vi "UMLEditor ToolBarSettings.vi"(1 "localVariables":T3 {"ObjectHotspots"."HotSpot"."y" format="%.2f"; "ObjectHotspots"."HotSpot"."x" format="%.2f"; "NodesBounds"."height" format="%.2f"; "NodesBounds"."width" format="%.2f"; "NodesBounds"."y" format="%.2f"; "NodesBounds"."x" format="%.2f"; "offset"."y" format="%.2f"; "offset"."x" format="%.2f"; "gridSize" format="%.2f"; "dragStartBounds"."height" format="%.2f"; "dragStartBounds"."width" format="%.2f"; "dragStartBounds"."y" format="%.2f"; "dragStartBounds"."x" format="%.2f"; "dragStartPoint"."y" format="%.2f"; "dragStartPoint"."x" format="%.2f"; "rubberBandStart"."y" format="%.2f"; "rubberBandStart"."x" format="%.2f"; "lastMousePoint"."y" format="%.2f"; "lastMousePoint"."x" format="%.2f"; "zoom" format="%.2f"}, 2 "NodeName/EdgeName(empty=not in use)":string, 3 "graph(only used with className input)":refnum<class "Graph.lvclass">, 5 "error in (no error)":errorcluster) -> (14 "diagramType":string, 15 "toolType":T2, 16 "tools":T1, 17 "prototypeEdge":refnum<class "AbstractEdge.lvclass">, 18 "prototypeNode":refnum<class "AbstractNode.lvclass">, 19 "error out":errorcluster)   [LabVIEW 2014]
doc: "Get Tollbar info\nif NodeName/EdgeName is used ..."
uses:
  <resource>/Framework/Providers/Open_GDS/UML/UMLEditor/UMLEditor LocalVariablesType.ctl
  <resource>/Framework/Providers/Open_GDS/UML/AbstractNode_class/AbstractNode.lvclass
  <resource>/Framework/Providers/Open_GDS/UML/AbstractEdge_class/AbstractEdge.lvclass
  <resource>/Framework/Providers/Open_GDS/UML/Graphics_class/Graphics.lvclass
  <resource>/Framework/Providers/Open_GDS/UML/Grid_class/Grid.lvclass
  <resource>/Framework/Providers/Open_GDS/UML/UMLEditor/UMLEditor statesType.ctl
  <resource>/Framework/Providers/Open_GDS/UML/UMLEditor/UMLEditor tooltype.ctl
  <resource>/Framework/Providers/Open_GDS/UML/UMLEditor/UMLEditor toolsType.ctl
  <resource>/Framework/Providers/Open_GDS/UML/UMLEditor/UMLEditor_DiagramInfo.ctl
  <resource>/Framework/Providers/Open_GDS/UML/Graph_class/Graph.lvclass
  <resource>/Framework/Providers/Open_GDS/UML/General/Point/Point Point2D.ctl
  <resource>/Framework/Providers/Open_GDS/UML/General/Rectangle/Rectangle Rectangle2D.ctl
  <resource>/Framework/Providers/Open_GDS/UML/UMLEditor/UMLEditor ExportType.ctl
  <resource>/Framework/Providers/Open_GDS/UML/UMLEditor/UMLEditor FlattenCommandType.ctl
  <resource>/Framework/Providers/Open_GDS/UML/UMLEditor/UMLEditor ExecuteCommandType.ctl
  <resource>/Framework/Providers/Open_GDS/UML/ContextHelp/ContextHelp_EventType.ctl
  <resource>/Framework/Providers/Open_GDS/UML/UMLEditor/UMLEditor_HotSpotData.ctl
  <resource>/Framework/Providers/Open_GDS/UML/UMLEditor/UMLEditor_HotSpotType.ctl
  <resource>/Framework/Providers/Open_GDS/UML/UmlEditor_class/EventData.ctl
  <resource>/Framework/Providers/Open_GDS/UML/UMLEditor/UMLEditor_DiagramType.ctl
  <resource>/Framework/Providers/Open_GDS/UML/UmlEditor_class/UmlEditor.lvclass
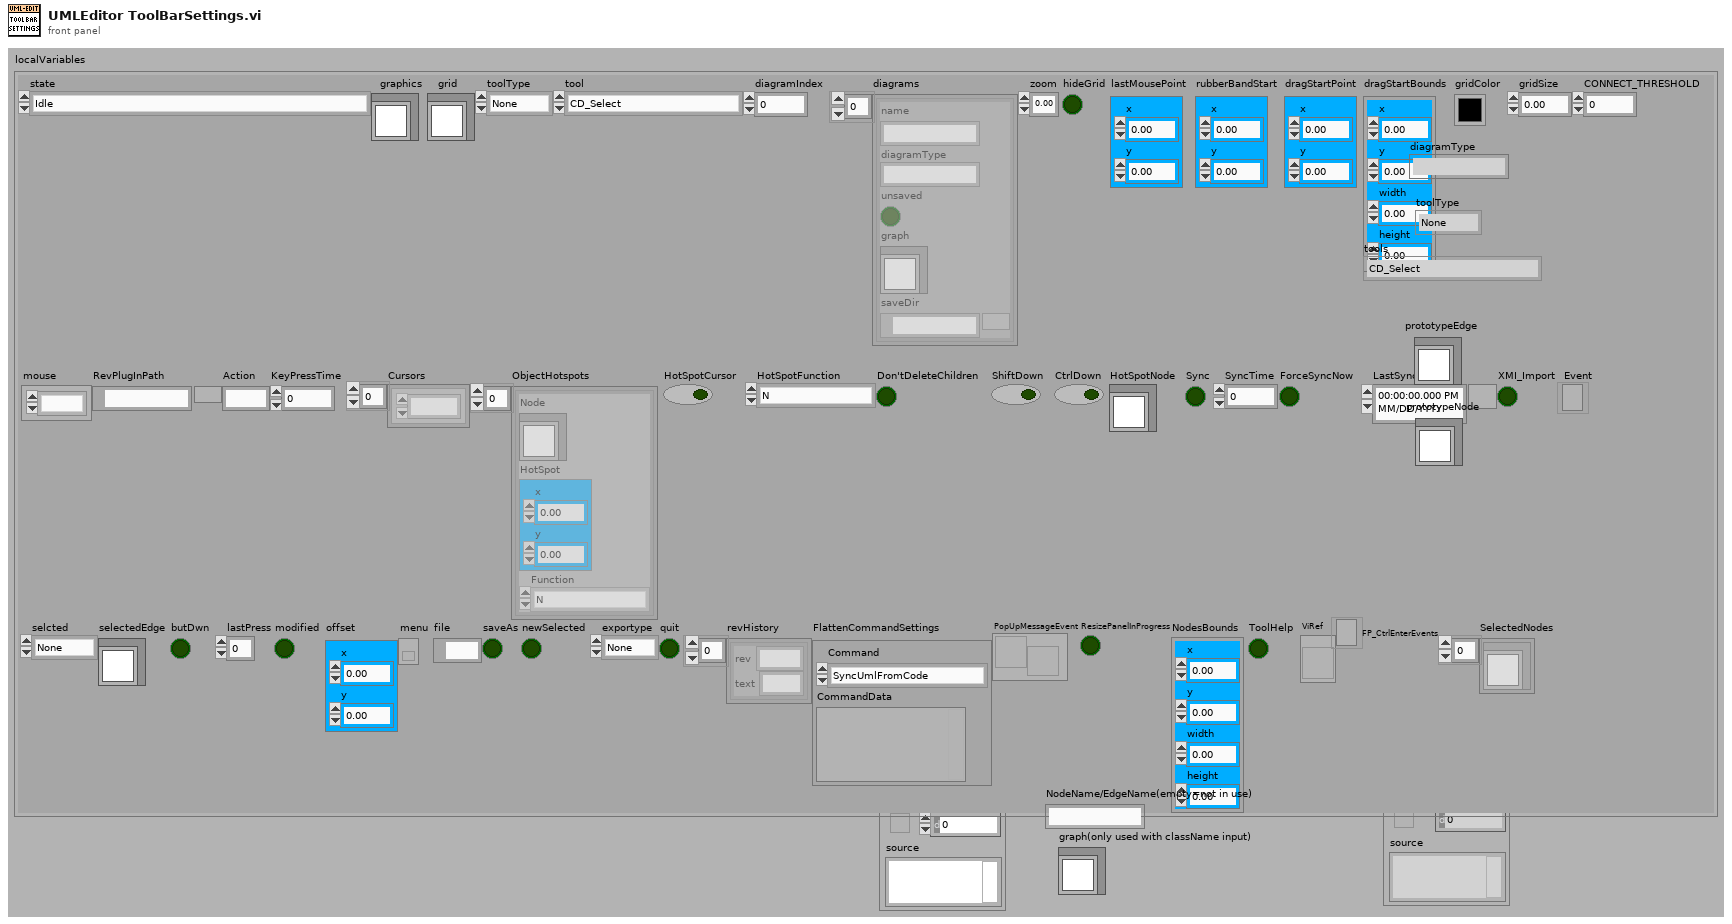
[diagram p1: front panel]
types:
  T1 = typedef "UMLEditor toolsType.ctl" = enum16{"CD_Select", "CD_Class", "CD_Interface", "CD_Package", "CD_Note", "CD_Dependency", "CD_Inheritance", "CD_InterfaceImp", "CD_Association", "CD_Aggregation", "CD_Composite", "CD_NoteConn", "SQD_Select", "SQD_Object", "SQD_ActionBar", "SQD_Note", "SQD_Call", "SQD_NoteConn", "UD_Select", "UD_System", "UD_Actor", "UD_UseCase", "UD_Note", "UD_Assoiciation", "UD_Generalization", "UD_GeneralizationIncludes", "UD_GeneralizationExtends", "UD_Realization", "UD_Relationship", "UD_NoteEdge", "STD_Select", "STD_State", "STD_InitailState", "STD_FinalState", "STD_ChoiseState", "STD_StateTransation", "STD_Note", "STD_NoteEdge", "DM_Select", "DM_VI", "DM_Module", "DM_Request", "DM_RequestWait", "DM_Roundtrip", "DM_Broadcast", "DM_Note", "DM_NoteEdge"}
  T2 = typedef "UMLEditor tooltype.ctl" = enum16{"None", "Node", "Edge"}
  T3 = typedef "UMLEditor LocalVariablesType.ctl" = cluster{"state":T4, "graphics":refnum<class "Graphics.lvclass">, "grid":refnum<class "Grid.lvclass">, "toolType":T2, "tool":T1, "diagramIndex":i32, "diagrams":T5[], "zoom":dbl, "hideGrid":bool, "lastMousePoint":T6, "rubberBandStart":T6, "dragStartPoint":T6, "dragStartBounds":T7, "gridColor":u32, "gridSize":dbl, "CONNECT_THRESHOLD":i32, "selcted":T2, "selectedEdge":refnum<class "AbstractEdge.lvclass">, "butDwn":bool, "lastPress":u32, "modified":bool, "offset":T6, "menu":refnum<k9>, "file":path, "saveAs":bool, "newSelected":bool, "exportype":T8, "quit":bool, "revHistory":cluster{"rev":string, "text":string}[], "FlattenCommandSettings":T9, "PopUpMessageEvent":T11, "ResizePanelInProgress":bool, "NodesBounds":T7, "ToolHelp":bool, "ViRef":refnum<vi>, "FP_CtrlEnterEvents":refnum<event-registration>, "SelectedNodes":refnum<class "AbstractNode.lvclass">[], "mouse":refnum<k1>, "RevPlugInPath":path, "Action":string, "KeyPressTime":u32, "Cursors":refnum<k1>[], "ObjectHotspots":T12[], "HotSpotCursor":bool, "HotSpotFunction":T13, "Don'tDeleteChildren":bool, "ShiftDown":bool, "CtrlDown":bool, "HotSpotNode":refnum<class "AbstractNode.lvclass">, "Sync":bool, "SyncTime":u32, "ForceSyncNow":bool, "LastSync":timestamp, "XMI_Import":bool, "Event":refnum<event-registration>}
  T4 = typedef "UMLEditor statesType.ctl" = enum16{"Idle", "CheckLicense", "revHistory", "Init", "Init2", "EditSelected", "RemoveSelected", "PaintComponent", "ChangeZoom", "ChangeGridSize", "Open", "Close", "Save", "ExportPicture", "Export", "Repaint", "Error", "Exit", "QUIT", "CreateScript", "ExecuteScript", "ClassReversedEngineering", "PlugInReverseEngineering", "StateReversedEngineering", "AutoPlace", "ExecuteCommand", "OpenClass", "SyncAll", "StraightenAssociation", "Copy", "Paste", "AddNodeFromProjectTree", "AddNodeFromProjectTree+SyncAll", "PanAndRepaint", "Init3", "CopyPaste", "ApplyDesignPattern", "AnalyseViInStateDiagram", "AutoSync"}
  T5 = typedef "UMLEditor_DiagramInfo.ctl" = cluster{"name":string, "diagramType":string, "unsaved":bool, "graph":refnum<class "Graph.lvclass">, "saveDir":path}
  T6 = typedef "Point Point2D.ctl" = cluster{"x":dbl, "y":dbl}
  T7 = typedef "Rectangle Rectangle2D.ctl" = cluster{"x":dbl, "y":dbl, "width":dbl, "height":dbl}
  T8 = typedef "UMLEditor ExportType.ctl" = enum16{"None", "Printer", "png", "jpg", "roseUML"}
  T9 = typedef "UMLEditor FlattenCommandType.ctl" = cluster{"Command":T10, "CommandData":variant}
  T10 = typedef "UMLEditor ExecuteCommandType.ctl" = enum16{"SyncUmlFromCode", "SyncCodeFromUML", "OpenClass", "OpenFile", "CreateClass", "CreateVI", "OpenClassAttribute", "LocateInProject"}
  T11 = typedef "ContextHelp_EventType.ctl" = refnum<user-event>
  T12 = typedef "UMLEditor_HotSpotData.ctl" = cluster{"Node":refnum<class "AbstractNode.lvclass">, "HotSpot":T6, "Function":T13}
  T13 = typedef "UMLEditor_HotSpotType.ctl" = enum16{"N", "NE", "E", "SE", "S", "SW", "W", "NW", "Expand", "Collaps"}
  T14 = typedef "UMLEditor_DiagramType.ctl" = string
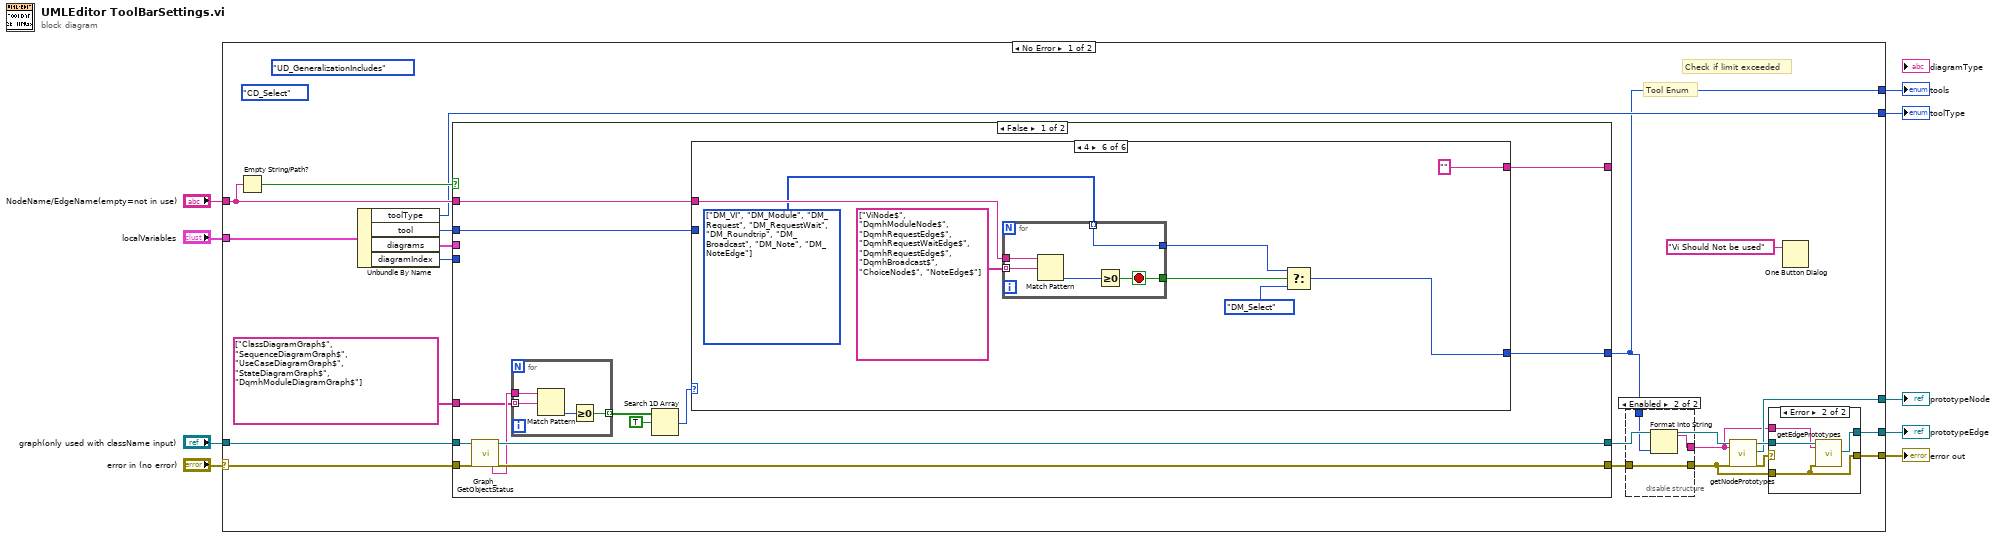
[diagram p0: block diagram]
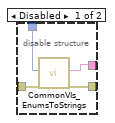
[diagram p2: hidden frame]
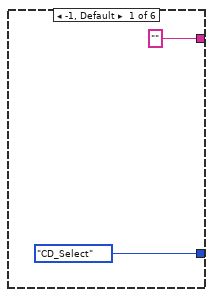
[diagram p4: hidden frame]
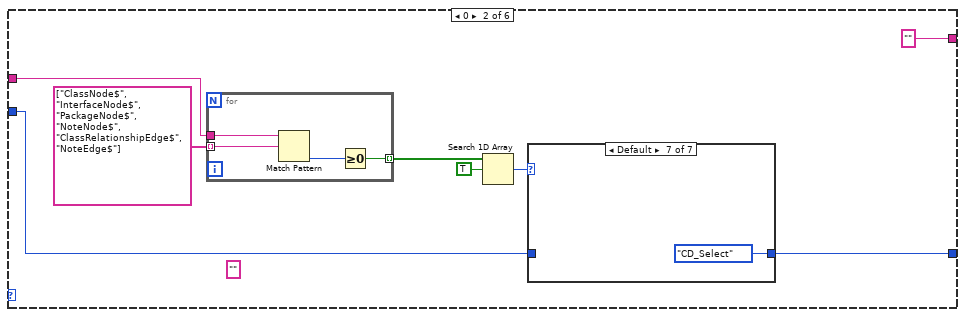
[diagram p5: hidden frame]
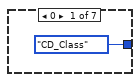
[diagram p6: hidden frame]
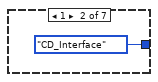
[diagram p7: hidden frame]
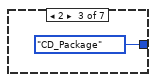
[diagram p8: hidden frame]
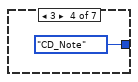
[diagram p9: hidden frame]
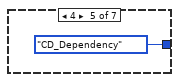
[diagram p10: hidden frame]
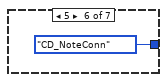
[diagram p11: hidden frame]
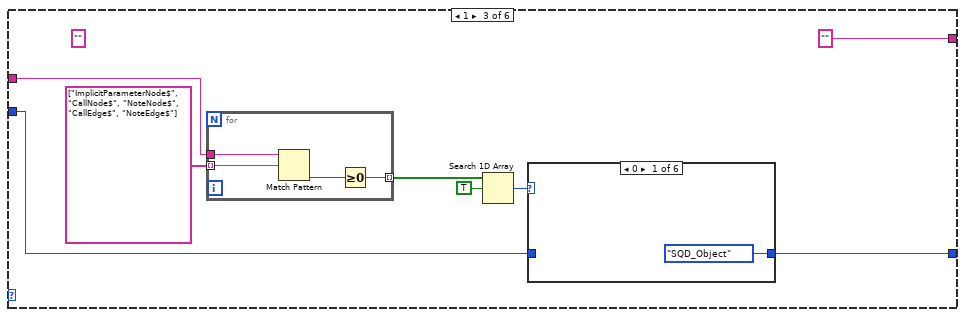
[diagram p12: hidden frame]
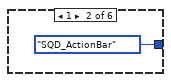
[diagram p13: hidden frame]
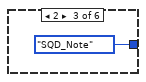
[diagram p14: hidden frame]
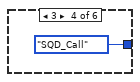
[diagram p15: hidden frame]
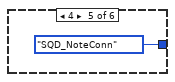
[diagram p16: hidden frame]
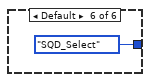
[diagram p17: hidden frame]
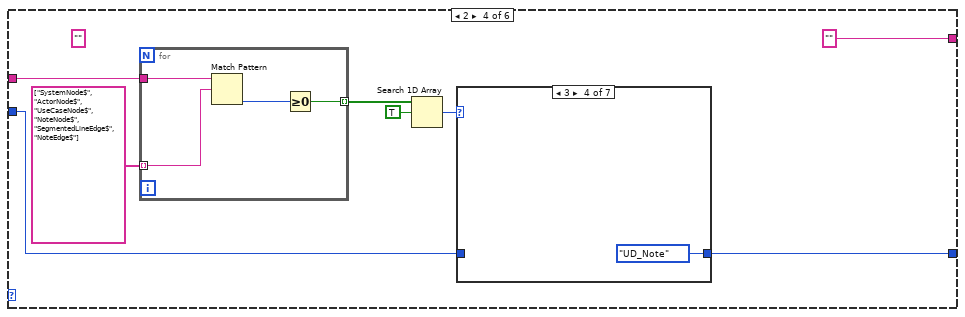
[diagram p18: hidden frame]
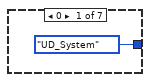
[diagram p19: hidden frame]
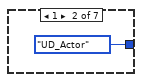
[diagram p20: hidden frame]
diagram:
  n1 = case shown="No Error" "error in (no error)" {
    selector: "error in (no error)" -> [w23 w156]
    tunnel: [w26 w156] -> w8
    tunnel: "localVariables" -> [w14 _]
    tunnel: [w19 _] -> w1
    tunnel: [w15 _] -> w6
    tunnel: [w12 _] -> w5
    tunnel: [w13 _] -> w4
    tunnel: "NodeName/EdgeName(empty=not in use)" -> [w21 _]
    tunnel: "graph(only used with className input)" -> [w24 _]
    frame No Error {
      (unwired) UMLEditor_toolsType."UD_GeneralizationIncludes" ("tool")
      (unwired) UMLEditor_toolsType."CD_Select" ("tool")
      # "Check if limit exceeded"
      # "Tool Enum"
      n2 = Empty String/Path?(string/path=w21) -> (empty?=w22:bool)
      n3 = Unbundle By Name(w14) -> ("toolType"=w13:T2, "tool"=w25:T1, "diagrams"=w30:T5[], "diagramIndex"=w29:i32)
      n4 = case shown="False" w22 {
        tunnel: w30 -> [_ w154]
        tunnel: w29 -> [_ w153]
        tunnel: [w50 w152] -> w28
        tunnel: [w45 _] -> _
        tunnel: w25 -> [w55 w151]
        tunnel: [w54 w151] -> w12
        tunnel: w24 -> [w53 _]
        tunnel: w23 -> [w52 w150]
        tunnel: [w51 w150] -> w18
        tunnel: w21 -> [w49 _]
        tunnel: string[] ["ClassDiagramGraph$", "SequenceDiagramGraph$", "UseCaseDiagramGraph$", "StateDiagramGraph$", "DqmhModuleDiagramGraph$"] -> [w47 _]
        frame False {
          n5 = call <resource>:"Graph_GetObjectStatus.vi"("reference in"=w53, "error in (no error)"=w52) -> ("Class name"=w48:string, "reference out"=w50:refnum<class "Graph.lvclass">, "error out"=w51:errorcluster)  [unwired: 15 out]
          n6 = for {
            tunnel: w48 -> [w149]
            tunnel: w47 -> [w148] mode=indexing
            tunnel: [w146] -> w44 mode=indexing
            n7 = Match Pattern(string=w149, regular expression=w148) -> (offset past match=w147:i32)  [unwired: 4 out]
            n8 = Greater Or Equal To 0?(x=w147) -> (x >= 0?=w146:bool)
          }
          n9 = Search 1D Array(1D array=w44, element=TRUE) -> (index of element=w46:i32)  [unwired: 1 out]
          n10 = case shown="4" w46 {
            tunnel: w55 -> [_ w65 w84 w102 w121 _]
            tunnel: [UMLEditor_toolsType."CD_Select" ("tool") w64 w83 w101 w120 w135] -> w54
            tunnel: w49 -> [_ w62 w81 w99 w118 w139]
            tunnel: [T14 "" ("diagramType") T14 "" ("diagramType") T14 "" ("diagramType") T14 "" ("diagramType") T14 "" ("diagramType") T14 "" ("diagramType")] -> w45
            frame -1, Default {
            }
            frame 0 {
              (unwired) T14 "" ("diagramType")
              n11 = for {
                tunnel: w62 -> [w69]
                tunnel: [w66] -> w59 mode=indexing
                tunnel: string[] ["ClassNode$", "InterfaceNode$", "PackageNode$", "NoteNode$", "ClassRelationshipEdge$", "NoteEdge$"] -> [w68] mode=indexing
                n12 = Match Pattern(string=w69, regular expression=w68) -> (offset past match=w67:i32)  [unwired: 4 out]
                n13 = Greater Or Equal To 0?(x=w67) -> (x >= 0?=w66:bool)
              }
              n14 = Search 1D Array(1D array=w59, element=TRUE) -> (index of element=w58:i32)  [unwired: 1 out]
              n15 = case shown="Default" w58 {
                tunnel: w65 -> [_ _ _ _ _ _ _]
                tunnel: [UMLEditor_toolsType."CD_Class" ("tool") UMLEditor_toolsType."CD_Interface" ("tool") UMLEditor_toolsType."CD_Package" ("tool") UMLEditor_toolsType."CD_Note" ("tool") UMLEditor_toolsType."CD_Dependency" ("tool") UMLEditor_toolsType."CD_NoteConn" ("tool") UMLEditor_toolsType."CD_Select" ("tool")] -> w64
                frame 0 {
                }
                frame 1 {
                }
                frame 2 {
                }
                frame 3 {
                }
                frame 4 {
                }
                frame 5 {
                }
                frame Default {
                }
              }
            }
            frame 1 {
              (unwired) T14 "" ("diagramType")
              n16 = for {
                tunnel: w81 -> [w88]
                tunnel: [w85] -> w78 mode=indexing
                tunnel: string[] ["ImplicitParameterNode$", "CallNode$", "NoteNode$", "CallEdge$", "NoteEdge$"] -> [w87] mode=indexing
                n17 = Match Pattern(string=w88, regular expression=w87) -> (offset past match=w86:i32)  [unwired: 4 out]
                n18 = Greater Or Equal To 0?(x=w86) -> (x >= 0?=w85:bool)
              }
              n19 = Search 1D Array(1D array=w78, element=TRUE) -> (index of element=w77:i32)  [unwired: 1 out]
              n20 = case shown="0" w77 {
                tunnel: w84 -> [_ _ _ _ _ _]
                tunnel: [UMLEditor_toolsType."SQD_Object" ("tool") UMLEditor_toolsType."SQD_ActionBar" ("tool") UMLEditor_toolsType."SQD_Note" ("tool") UMLEditor_toolsType."SQD_Call" ("tool") UMLEditor_toolsType."SQD_NoteConn" ("tool") UMLEditor_toolsType."SQD_Select" ("tool")] -> w83
                frame 0 {
                }
                frame 1 {
                }
                frame 2 {
                }
                frame 3 {
                }
                frame 4 {
                }
                frame Default {
                }
              }
            }
            frame 2 {
              (unwired) T14 "" ("diagramType")
              n21 = for {
                tunnel: w99 -> [w106]
                tunnel: [w103] -> w96 mode=indexing
                tunnel: string[] ["SystemNode$", "ActorNode$", "UseCaseNode$", "NoteNode$", "SegmentedLineEdge$", "NoteEdge$"] -> [w105] mode=indexing
                n22 = Match Pattern(string=w106, regular expression=w105) -> (offset past match=w104:i32)  [unwired: 4 out]
                n23 = Greater Or Equal To 0?(x=w104) -> (x >= 0?=w103:bool)
              }
              n24 = Search 1D Array(1D array=w96, element=TRUE) -> (index of element=w95:i32)  [unwired: 1 out]
              n25 = case shown="3" w95 {
                tunnel: w102 -> [_ _ _ _ _ _ _]
                tunnel: [UMLEditor_toolsType."UD_System" ("tools") UMLEditor_toolsType."UD_Actor" ("tools") UMLEditor_toolsType."UD_UseCase" ("tools") UMLEditor_toolsType."UD_Note" ("tools") UMLEditor_toolsType."UD_Assoiciation" ("tools") UMLEditor_toolsType."UD_NoteEdge" ("tools") UMLEditor_toolsType."UD_Select" ("tool")] -> w101
                frame 0 {
                }
                frame 1 {
                }
                frame 2 {
                }
                frame 3 {
                }
                frame 4 {
                }
                frame 5 {
                }
                frame Default {
                }
              }
            }
            frame 3 {
              (unwired) T14 "" ("diagramType")
              # "NOT IS USE???"
              n26 = for {
                tunnel: w118 -> [w125]
                tunnel: [w122] -> w115 mode=indexing
                tunnel: string[] ["FinalStateNode$", "InitialStateNode$", "StateNode$", "StateTransitionEdge$", "NoteNode$", "NoteEdge$", "ChoiceNode$"] -> [w124] mode=indexing
                n27 = Match Pattern(string=w125, regular expression=w124) -> (offset past match=w123:i32)  [unwired: 4 out]
                n28 = Greater Or Equal To 0?(x=w123) -> (x >= 0?=w122:bool)
              }
              n29 = Search 1D Array(1D array=w115, element=TRUE) -> (index of element=w114:i32)  [unwired: 1 out]
              n30 = case shown="Default" w114 {
                tunnel: w121 -> [_ _ _ _ _ _ _]
                tunnel: [UMLEditor_toolsType."STD_FinalState" ("tools") UMLEditor_toolsType."STD_InitailState" ("tools") UMLEditor_toolsType."STD_State" ("tools") UMLEditor_toolsType."STD_StateTransation" ("tools") UMLEditor_toolsType."STD_Note" ("tools") UMLEditor_toolsType."STD_NoteEdge" ("tools") UMLEditor_toolsType."STD_ChoiseState" ("tools")] -> w120
                frame 0 {
                }
                frame 1 {
                }
                frame 2 {
                }
                frame 3 {
                }
                frame 4 {
                }
                frame Default {
                }
                frame 6 {
                }
              }
            }
            frame 4 {
              w134 = T1[] [enum."DM_VI", enum."DM_Module", enum."DM_Request", enum."DM_RequestWait", enum."DM_Roundtrip", enum."DM_Broadcast", enum."DM_Note", enum."DM_NoteEdge"] items=["CD_Select", "CD_Class", "CD_Interface", "CD_Package", "CD_Note", "CD_Dependency", "CD_Inheritance", "CD_InterfaceImp", "CD_Association", "CD_Aggregation", "CD_Composite", "CD_NoteConn", "SQD_Select", "SQD_Object", "SQD_ActionBar", "SQD_Note", "SQD_Call", "SQD_NoteConn", "UD_Select", "UD_System", "UD_Actor", "UD_UseCase", "UD_Note", "UD_Assoiciation", "UD_Generalization", "UD_GeneralizationIncludes", "UD_GeneralizationExtends", "UD_Realization", "UD_Relationship", "UD_NoteEdge", "STD_Select", "STD_State", "STD_InitailState", "STD_FinalState", "STD_ChoiseState", "STD_StateTransation", "STD_Note", "STD_NoteEdge", "DM_Select", "DM_VI", "DM_Module", "DM_Request", "DM_RequestWait", "DM_Roundtrip", "DM_Broadcast", "DM_Note", "DM_NoteEdge"]
              n31 = for {
                tunnel: w139 -> [w145]
                tunnel: [w142] -> w137
                tunnel: string[] ["ViNode$", "DqmhModuleNode$", "DqmhRequestEdge$", "DqmhRequestWaitEdge$", "DqmhRequestEdge$", "DqmhBroadcast$", "ChoiceNode$", "NoteEdge$"] -> [w144] mode=indexing
                tunnel: [w141] -> w133
                tunnel: w134 -> [w141] mode=indexing
                stop <- w142 stop-if-true
                n32 = Match Pattern(string=w145, regular expression=w144) -> (offset past match=w143:i32)  [unwired: 4 out]
                n33 = Greater Or Equal To 0?(x=w143) -> (x >= 0?=w142:bool)
              }
              n34 = Select(t=w133, s=w137, f=UMLEditor_toolsType."DM_Select" ("tools")) -> (s? t:f=w135:T1)
            }
          }
        }
        frame True {
          n35 = Index Array(array=w154, index=w153) -> (element=w155:T5)
          n36 = Unbundle By Name(w155) -> ("graph"=w152:refnum<class "Graph.lvclass">)  [unwired: 1 out]
        }
      }
      n37 = disable-structure shown="Enabled" {
        disable-tunnel: w18 -> [w34 w35]
        disable-tunnel: [w33 w35] -> w16
        disable-tunnel: w12 -> [w32 w37]
        disable-tunnel: [w31 w36] -> w11
        frame Disabled {
          n38 = call <resource>:"CommonVIs_EnumsToStrings.vi"("SingleEnumVariantIn"=w32, "error in (no error)"=w34) -> ("EnumItem"=w31:string, "error out"=w33:errorcluster)  [unwired: 1 in, 15 out]
        }
        frame Enabled {
          n39 = Format Into String(w37) -> (resulting string=w36:string)  [unwired: 3 in, 1 out]
        }
      }
      n40 = call-dynamic "getNodePrototypes.vi"("reference"=w28, "NodeName"=w11, "error in (no error)"=w16) -> ("reference out"=w27:refnum<class "Graph.lvclass">, "node"=w19:refnum<class "AbstractNode.lvclass">, "error out"=w17:errorcluster)  [unwired: 13 in, 1 out]
      n41 = case shown="Error" w17 {
        selector: w17 -> [w38 _]
        tunnel: w27 -> [_ w42]
        tunnel: [w38 w39] -> w26
        tunnel: w16 -> [_ w39]
        tunnel: [_ w41] -> w15
        tunnel: w11 -> [_ w40]
        frame No Error {
        }
        frame Error {
          n42 = call-dynamic "getEdgePrototypes.vi"("reference"=w42, "EdgeName"=w40, "error in (no error)"=w39) -> ("edge"=w41:refnum<class "AbstractEdge.lvclass">)  [unwired: 13 in, 3 out]
        }
      }
      n43 = One Button Dialog(message="Vi Should Not be used") -> ()  [unwired: 1 in, 1 out]
    }
    frame Error {
    }
  }
  "error out" <- w8
  "prototypeNode" <- w1
  "prototypeEdge" <- w6
  "tools" <- w5
  "toolType" <- w4
